vi "Day 14 Amicable pairs.vi"() -> ()   [LabVIEW 2026]
panel:
  out "Discovered Amicable Numbers List":i32[](array[numeric])
  in  "Search Upper Limit":i32
  out "Is Amicable Pairs":bool
  out "sum B":i32
  out "sum A":i32
  out "Array B":i32[](array[numeric])
  in  "B":i32
  out "Array A":i32[](array[numeric])
  in  "A":i32
  out "The Perfect Number???":bool
  out "sum":i32
  out "Array":i32[](array[numeric])
  in  "Numeric":i32
  # "Check whether one number is “perfect” (equals the sum of its proper divisors)"
  # "Check whether one number is “perfect” (equals the sum of its proper divisors)"
  # "Find and list all amicable pairs below a user-specified limit"
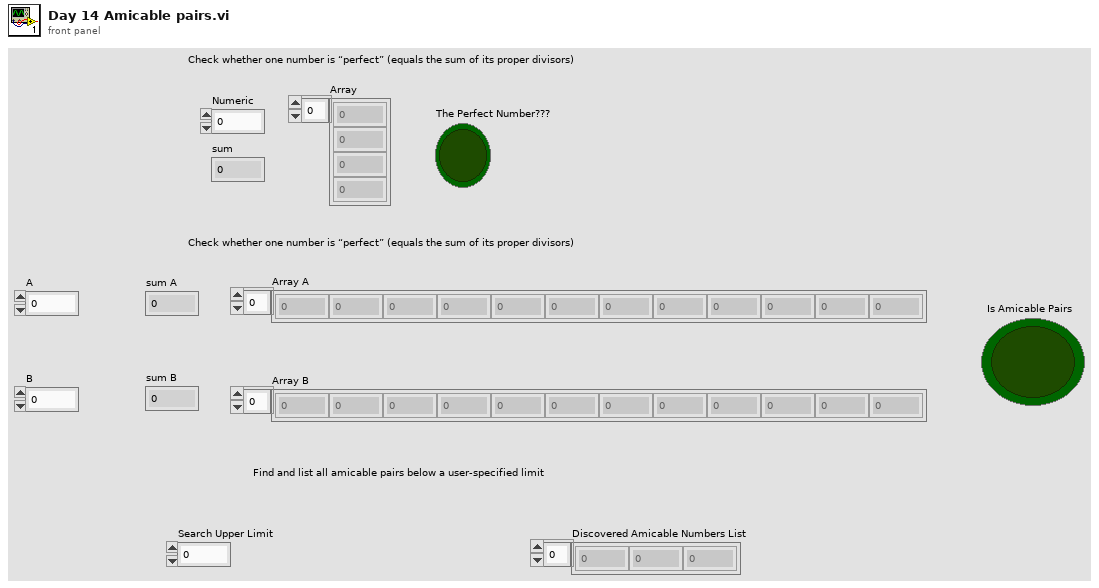
[diagram p1: front panel]
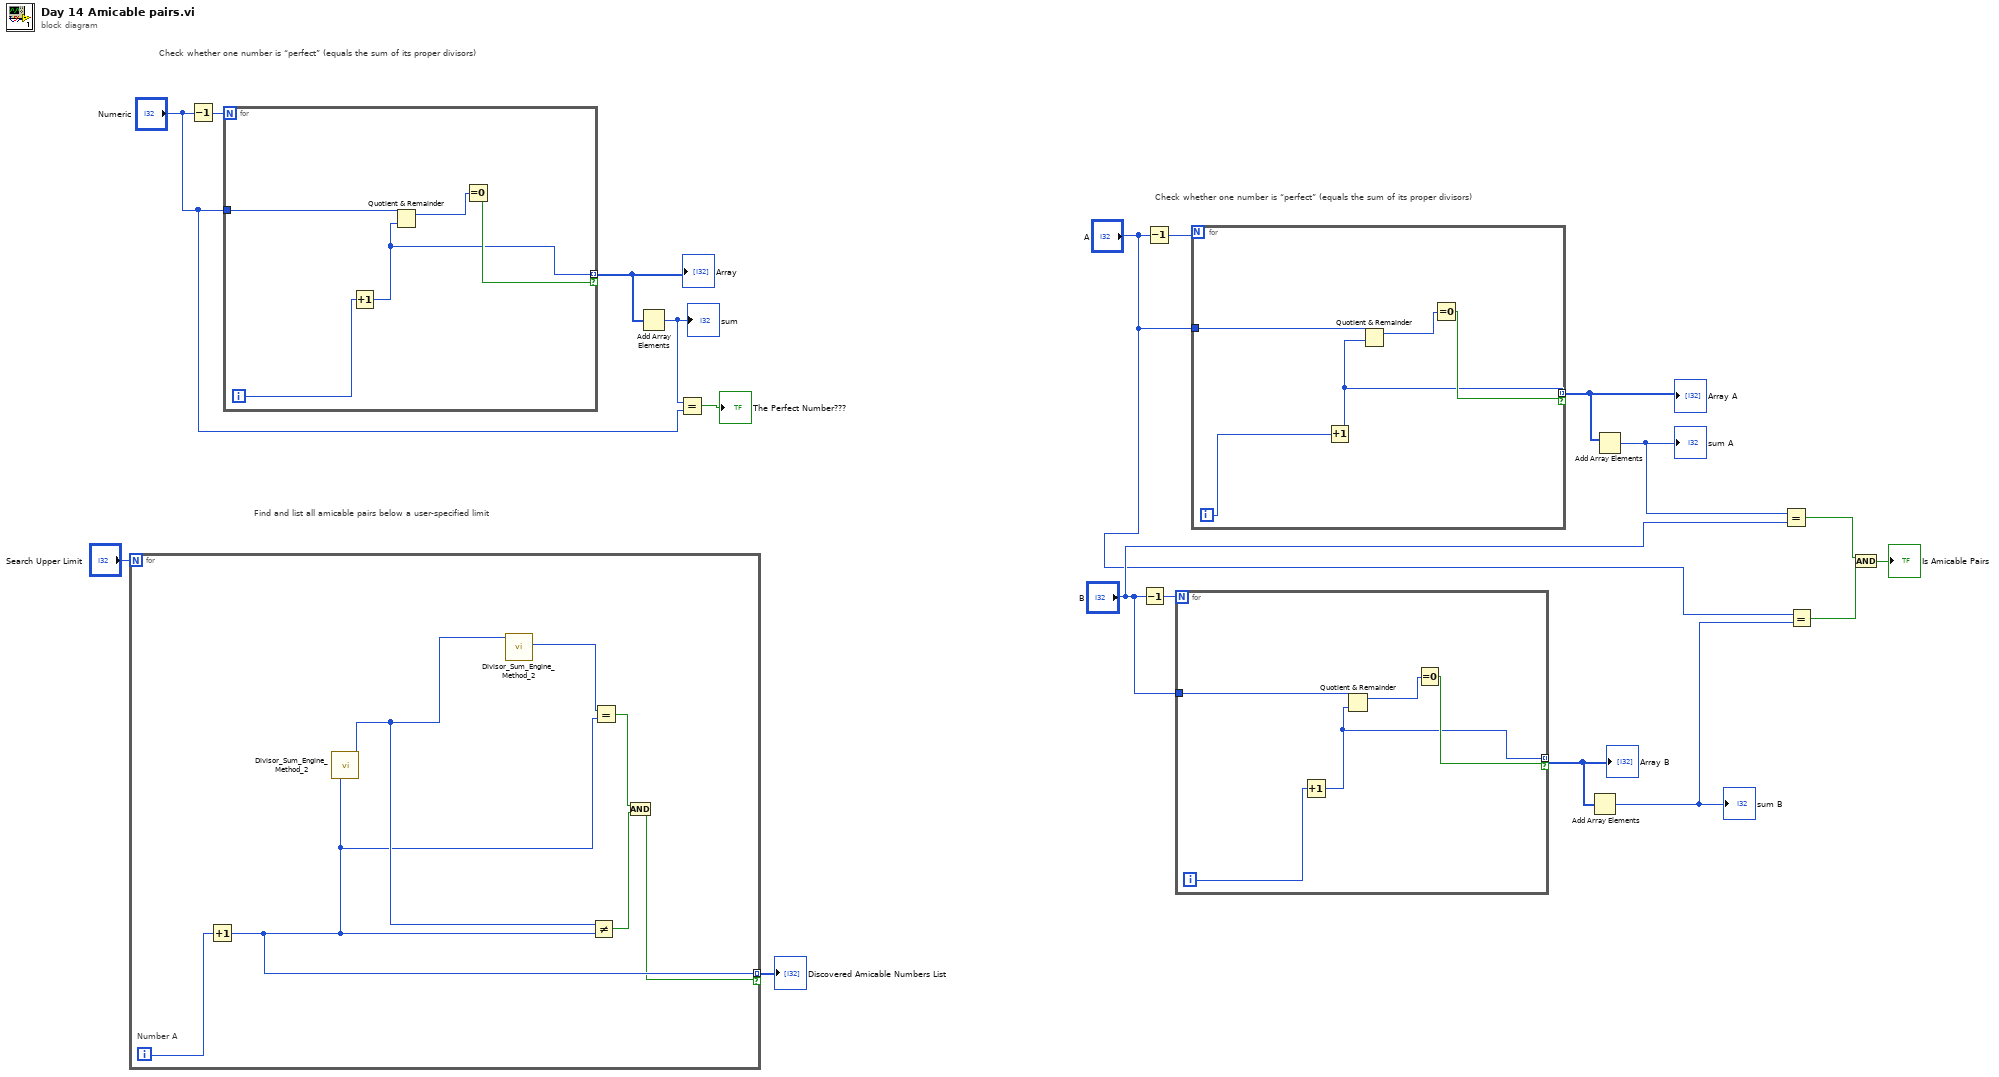
[diagram p0: block diagram]
diagram:
  # "Check whether one number is “perfect” (equals the sum of its proper divisors)"
  # "Check whether one number is “perfect” (equals the sum of its proper divisors)"
  # "Find and list all amicable pairs below a user-specified limit"
  n1 = for {
    N: "Search Upper Limit" -> [_]
    tunnel: [w22] -> w1 mode=indexing if=w19
    i -> [w25]
    # "Number A"
    n2 = Increment(x=w25) -> (x+1=w22:i32)
    n3 = call "Divisor_Sum_Engine_Method_2.vi"("N"=w22) -> ("Numeric"=w23:i32)  [unwired: 9 in, 1 out]
    n4 = call "Divisor_Sum_Engine_Method_2.vi"("N"=w23) -> ("Numeric"=w24:i32)  [unwired: 9 in, 1 out]
    n5 = Not Equal?(x=w23, y=w22) -> (x != y?=w20:bool)
    n6 = Equal?(x=w24, y=w22) -> (x = y?=w21:bool)
    n7 = And(x=w21, y=w20) -> (x .and. y?=w19:bool)
  }
  "Discovered Amicable Numbers List" <- w1
  n8 = Decrement(x="Numeric") -> (x-1=w18:i32)
  n9 = for {
    N: w18 -> [_]
    tunnel: "Numeric" -> [w29]
    tunnel: [w26] -> w17 mode=indexing if=w28
    i -> [w27]
    n10 = Increment(x=w27) -> (x+1=w26:i32)
    n11 = Quotient & Remainder(x=w29, y=w26) -> (x-y*floor(x/y)=w30:i32)  [unwired: 1 out]
    n12 = Equal To 0?(x=w30) -> (x = 0?=w28:bool)
  }
  "Array" <- w17
  n13 = Add Array Elements(numeric array=w17) -> (sum=w16:i32)
  "sum" <- w16
  n14 = Equal?(x=w16, y="Numeric") -> (x = y?=→"The Perfect Number???":bool)
  n15 = Decrement(x="B") -> (x-1=w12:i32)
  n16 = Decrement(x="A") -> (x-1=w13:i32)
  n17 = for {
    N: w12 -> [_]
    tunnel: "B" -> [w34]
    tunnel: [w31] -> w11 mode=indexing if=w33
    i -> [w32]
    n18 = Increment(x=w32) -> (x+1=w31:i32)
    n19 = Quotient & Remainder(x=w34, y=w31) -> (x-y*floor(x/y)=w35:i32)  [unwired: 1 out]
    n20 = Equal To 0?(x=w35) -> (x = 0?=w33:bool)
  }
  "Array B" <- w11
  n21 = for {
    N: w13 -> [_]
    tunnel: "A" -> [w39]
    tunnel: [w36] -> w3 mode=indexing if=w38
    i -> [w37]
    n22 = Increment(x=w37) -> (x+1=w36:i32)
    n23 = Quotient & Remainder(x=w39, y=w36) -> (x-y*floor(x/y)=w40:i32)  [unwired: 1 out]
    n24 = Equal To 0?(x=w40) -> (x = 0?=w38:bool)
  }
  "Array A" <- w3
  n25 = Add Array Elements(numeric array=w11) -> (sum=w8:i32)
  "sum B" <- w8
  n26 = Add Array Elements(numeric array=w3) -> (sum=w10:i32)
  "sum A" <- w10
  n27 = Equal?(x=w10, y="B") -> (x = y?=w6:bool)
  n28 = Equal?(x="A", y=w8) -> (x = y?=w5:bool)
  n29 = And(x=w6, y=w5) -> (x .and. y?=→"Is Amicable Pairs":bool)
